vi "SEA_CURRENT_CONTROL_PI.vi"() -> ()   [LabVIEW 2019]
uses:
  <vilib>/rvi/Emulation/niFpgaGetClockAttributes.vi
  <vilib>/rvi/Emulation/niFpgaSctlEmulationGetInTimedLoop.vi
  <vilib>/rvi/Emulation/niFpgaEmulationReportErrorSimple.vi
  <vilib>/rvi/eio/common/nirviEmuTemplateMethod_errors.vi
  <vilib>/rvi/Emulation/niFpgaCriticalErrorInLSC.vi
  <vilib>/eio/EIONode/EIONode.xnode
panel:
  out "Loop rate":u32
  out "filtered current":sgl
  in  "Reference":sgl
  in  "Ki":sgl
  out "Motor Direction":bool
  in  "LB":sgl
  in  "UB":sgl
  in  "Kp":sgl
  in  "Current Offset":sgl=2.4882812 format="%#_13g"
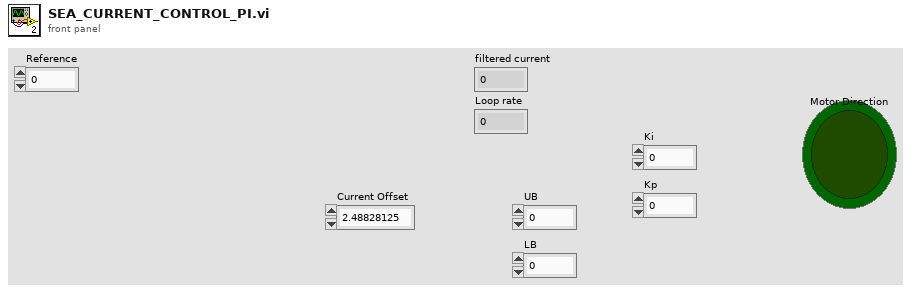
[diagram p1: front panel]
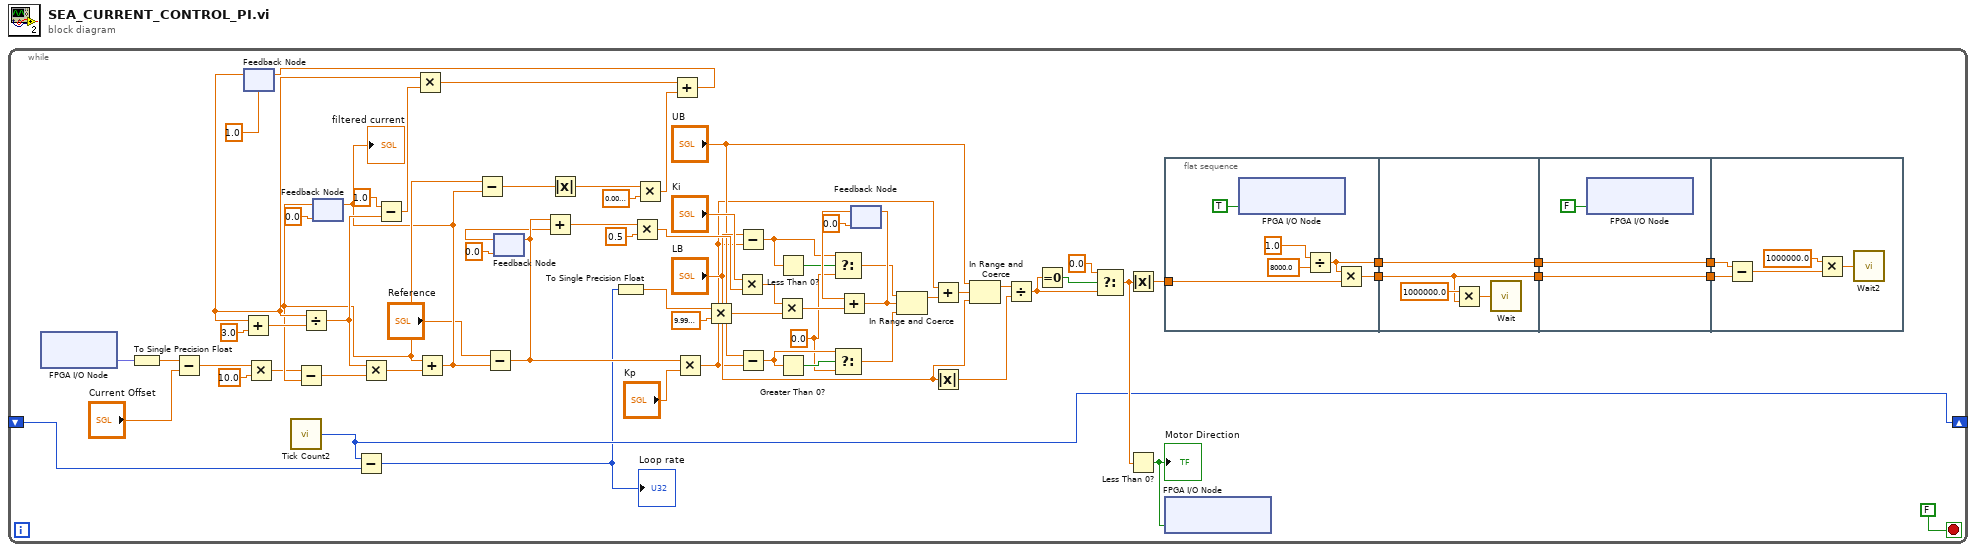
[diagram p0: block diagram]
diagram:
  n1 = while {
    shift-right: [w3] -> _
    shift-left: _ -> [w2]
    stop <- FALSE stop-if-true
    w14 = sgl 0.0 ("f")
    n2 = xnode "FPGA I/O Node"() -> ("AI9"=w6:fxp<+/-,24,5>)  [unwired: 1 in, 1 out]
    n3 = To Single Precision Float(number=w6) -> (single precision float=w5:sgl)
    n4 = Subtract(x=w5, y="Current Offset") -> (x-y=w45:sgl)
    n5 = feedback #1(sgl 1.0) -> (w56:sgl)
    n6 = Add(x=w56, y=sgl 3.0) -> (x+y=w65:sgl)
    n7 = Multiply(x=w45, y=sgl 10.0) -> (x*y=w47:sgl)
    n8 = call "Tick Count2"() -> ("Tick Count(uSec)"=w3:u32)
    n9 = Divide(x=w56, y=w65) -> (x/y=w62:sgl)
    n10 = feedback #2(sgl 0.0) -> (w55:sgl)
    n11 = Subtract(x=w47, y=w55) -> (x-y=w63:sgl)
    n12 = Subtract(x=w3, y=w2) -> (x-y=w1:u32)
    "Loop rate" <- w1
    n13 = Multiply(x=w62, y=w63) -> (x*y=w64:sgl)
    n14 = Subtract(x=sgl 1.0, y=w62) -> (x-y=w61:sgl)
    n15 = Multiply(x=w56, y=w61) -> (x*y=w60:sgl)
    n16 = Add(x=w55, y=w64) -> (x+y=w8:sgl)
    "filtered current" <- w8
    n17 = feedback-in #2(w8) -> ()
    n18 = Subtract(x=w55, y=w8) -> (x-y=w59:sgl)
    n19 = Subtract(x="Reference", y=w8) -> (x-y=w35:sgl)
    n20 = feedback-in #3(w35) -> ()
    n21 = feedback #3(sgl 0.0) -> (w34:sgl)
    n22 = Add(x=w35, y=w34) -> (x+y=w33:sgl)
    n23 = Absolute Value(x=w59) -> (abs(x)=w58:sgl)
    n24 = To Single Precision Float(number=w1) -> (single precision float=w25:sgl)
    n25 = Multiply(x=w33, y=sgl 0.5) -> (x*y=w31:sgl)
    n26 = Multiply(x=w58, y=sgl 0.01) -> (x*y=w57:sgl)
    n27 = Add(x=w60, y=w57) -> (x+y=w49:sgl)
    n28 = feedback-in #1(w49) -> ()
    n29 = Multiply(x=w35, y="Kp") -> (x*y=w17:sgl)
    n30 = Multiply(x=w25, y=sgl 1e-06) -> (x*y=w23:sgl)
    n31 = Multiply(x="Ki", y=w31) -> (x*y=w26:sgl)
    n32 = Subtract(x="LB", y=w17) -> (x-y=w19:sgl)
    n33 = Subtract(x="UB", y=w17) -> (x-y=w15:sgl)
    n34 = Multiply(x=w26, y=w23) -> (x*y=w22:sgl)
    n35 = Less Than 0?(x=w19) -> (x < 0?=w20:bool)
    n36 = Greater Than 0?(x=w15) -> (x > 0?=w16:bool)
    n37 = Select(t=w19, s=w20, f=w14) -> (s? t:f=w12:sgl)
    n38 = Select(t=w15, s=w16, f=w14) -> (s? t:f=w11:sgl)
    n39 = feedback #4(sgl 0.0) -> (w28:sgl)
    n40 = Add(x=w28, y=w22) -> (x+y=w13:sgl)
    n41 = feedback-in #4(w13) -> ()
    n42 = In Range and Coerce(upper limit=w12, x=w13, lower limit=w11) -> (coerced(x)=w10:sgl)  [unwired: 1 out]
    n43 = Add(x=w17, y=w10) -> (x+y=w27:sgl)
    n44 = Absolute Value(x="LB") -> (abs(x)=w42:sgl)
    n45 = In Range and Coerce(upper limit="UB", x=w27, lower limit="LB") -> (coerced(x)=w43:sgl)  [unwired: 1 out]
    n46 = Divide(x=w43, y=w42) -> (x/y=w39:sgl)
    n47 = Equal To 0?(x=w39) -> (x = 0?=w41:bool)
    n48 = Select(t=sgl 0.0, s=w41, f=w39) -> (s? t:f=w37:sgl)
    n49 = Absolute Value(x=w37) -> (abs(x)=w4:sgl)
    n50 = Less Than 0?(x=w37) -> (x < 0?=w38:bool)
    "Motor Direction" <- w38
    n51 = flat-sequence {
      tunnel: [w76] -> w71
      tunnel: [w74] -> w70
      tunnel: w4 -> [w72]
      tunnel: w71 -> [w79]
      tunnel: [w79] -> w69
      tunnel: w70 -> [w78]
      tunnel: [w78] -> w68
      tunnel: w69 -> [w84]
      tunnel: [w84] -> w67
      tunnel: w68 -> [w83]
      tunnel: [w83] -> w66
      tunnel: w67 -> [w89]
      tunnel: w66 -> [w85]
      frame #0 {
        n52 = xnode "FPGA I/O Node"("RMC/DIO33"=TRUE) -> ()  [unwired: 1 in, 1 out]
        n53 = Divide(x=sgl 1.0, y=sgl 8000.0) -> (x/y=w74:sgl)
        n54 = Multiply(x=w74, y=w72) -> (x*y=w76:sgl)
      }
      frame #1 {
        n55 = Multiply(x=sgl 1000000.0, y=w79) -> (x*y=w81:sgl)
        n56 = call "Wait"("Count(uSec)"=w81) -> ()  [unwired: 1 out]
      }
      frame #2 {
        n57 = xnode "FPGA I/O Node"("RMC/DIO33"=FALSE) -> ()  [unwired: 1 in, 1 out]
      }
      frame #3 {
        n58 = Subtract(x=w85, y=w89) -> (x-y=w88:sgl)
        n59 = Multiply(x=sgl 1000000.0, y=w88) -> (x*y=w87:sgl)
        n60 = call "Wait2"("Count(uSec)"=w87) -> ()  [unwired: 1 out]
      }
    }
    n61 = xnode "FPGA I/O Node"("RMC/DIO34"=w38) -> ()  [unwired: 1 in, 1 out]
  }
